vi "Set SG Path.vi"(0 "Path in":refnum<class "Scalar Path.lvclass">, 5 "Cal point in":T1, 11 "error in (no error)":errorcluster) -> (4 "Path out":refnum<class "Scalar Path.lvclass">, 6 "Cal point out":T1, 8 "Source Gain":dbl, 10 "Digital Gain":dbl, 15 "error out":errorcluster)   [LabVIEW 2023, in "RFFixtureCharact.Public.lvlib" / "Scalar Path.lvclass"]
uses:
  Scalar Path.lvclass
  Type Definitions/Cal Point.ctl
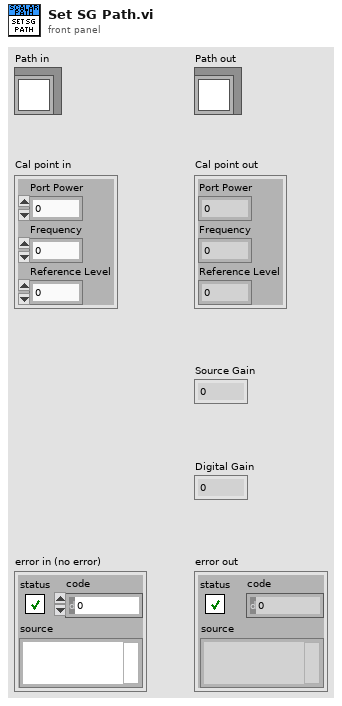
[diagram p1: front panel]
types:
  T1 = typedef "RFFixtureCharact.Public.lvlib/Scalar Path.lvclass/Cal Point.ctl" = cluster{"Port Power":dbl, "Frequency":dbl, "Reference Level":dbl}
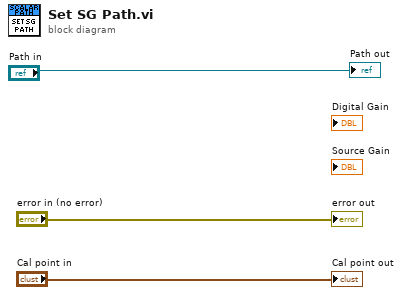
[diagram p0: block diagram]
diagram:
  "error out" <- "error in (no error)"
  "Cal point out" <- "Cal point in"
  "Path out" <- "Path in"
